vi "XDataNode_OnFontChange.vi"(0 "XRef":T10, 1 "State In":T1 {"Timing"."I/O Scan Engine Mode" max=255 format="%#.0f"; "Timing"."Assigned CPU" min=-2 max=255 format="%#.0f"}) -> (14 "Reply":T8, 15 "State Out":T1 {"Timing"."I/O Scan Engine Mode" max=255 format="%#.0f"; "Timing"."Assigned CPU" min=-2 max=255 format="%#.0f"})   [LabVIEW 2017, in "XDataNode.xnode"]
uses:
  XDataNode.xnode
  XNodeXNodeRef.ctl
  XDataNode.ctl
  timing_clust.ctl
  nitl_modes.ctl
  wakeup.ctl
  TermInfo.ctl
  nitl_TargetSpecificData.ctl
  DN_Type.ctl
  XNodeStringArray.ctl
  XNodeString.ctl
  ReplySet.ctl
  NI_XNodeSupport.lvlib
  XDNodeRunTimeDep.lvlib
panel:
  # "Expected End [f-1]"
  # "Actual End [f-1]"
  # "Finished Late? [f-1]"
  # "Expected End [i-1]"
  # "Actual End [i-1]"
  # "Finished Late? [i-1]"
  # "Exp.Iter.Start"
  # "Act.Iter.Start"
  # "Exp.Frm.Start"
  # "Act.Frm.Start"
  # "Source Name"
  # "Loop/Sequence Name"
  # "Period"
  # "Deadline"
  # "Offset"
  # "Start"
  # "Priority"
  # "Timeout"
  # "Mode"
  # "Wakeup Reason"
  # "Error"
  # "Source Type"
  # "2nd.Src.Type"
  # "Global End Time"
  # "Global Start Time"
  # "Frame Duration"
  # "Iteration Duration"
  # "Assigned CPU"
  # "I/O Scan Engine Mode"
  # "Expected End [f-1]"
  # "Actual End [f-1]"
  # "Finished Late? [f-1]"
  # "Expected End [i-1]"
  # "Actual End [i-1]"
  # "Finished Late? [i-1]"
  # "Exp.Iter.Start"
  # "Act.Iter.Start"
  # "Exp.Frm.Start"
  # "Act.Frm.Start"
  # "Source Name"
  # "Loop/Sequence Name"
  # "Period"
  # "Deadline"
  # "Offset"
  # "Start"
  # "Priority"
  # "Timeout"
  # "Mode"
  # "Wakeup Reason"
  # "Error"
  # "Source Type"
  # "2nd.Src.Type"
  # "Global End Time"
  # "Global Start Time"
  # "Frame Duration"
  # "Iteration Duration"
  # "Assigned CPU"
  # "I/O Scan Engine Mode"
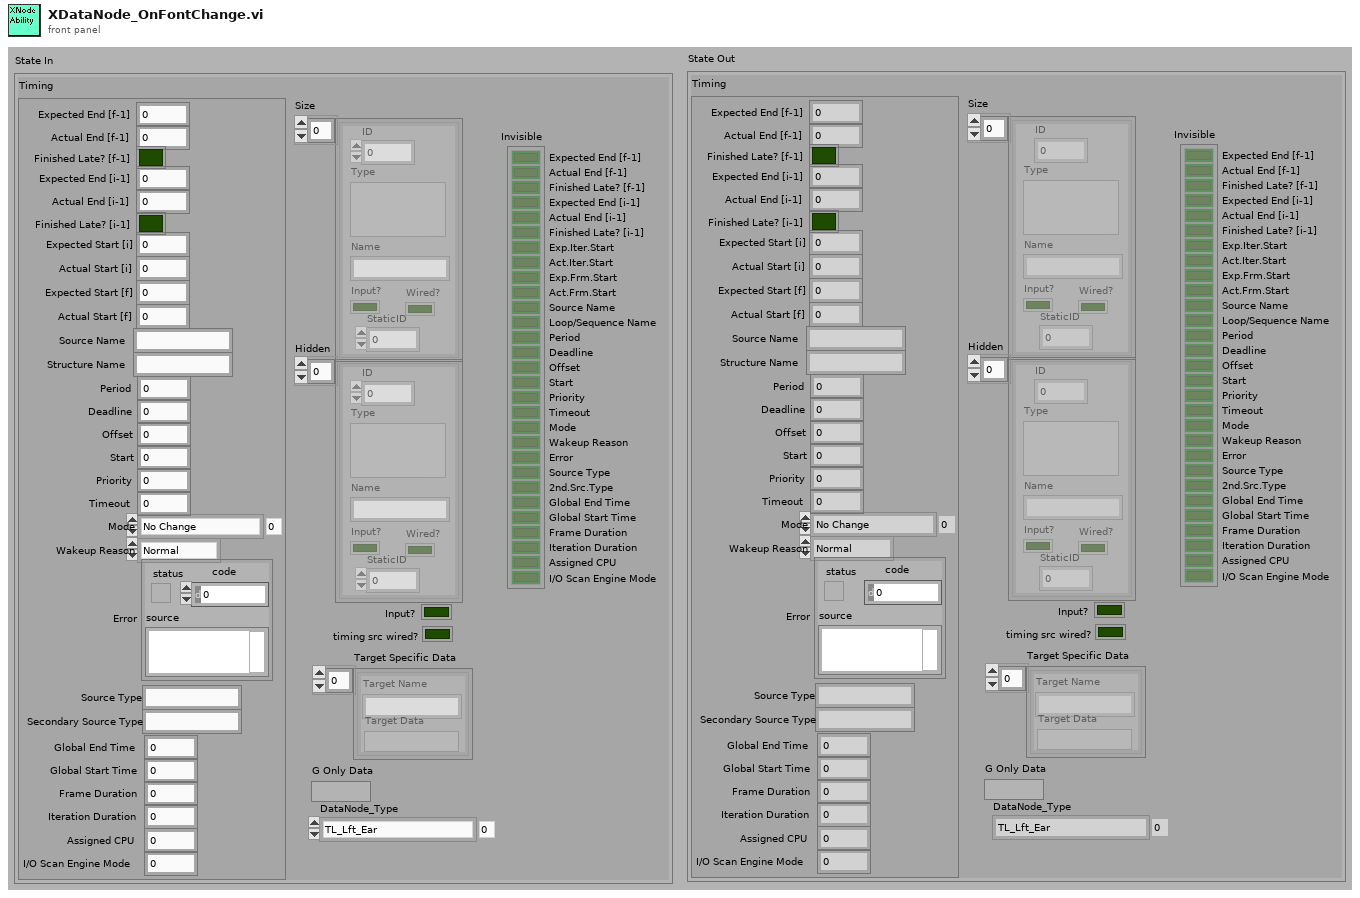
[diagram p1: front panel]
types:
  T1 = typedef "XDataNode.xnode/XDataNode.ctl" = cluster{"Timing":T2, "Size":T5[], "Hidden":T5[], "Invisible":bool[], "Input?":bool, "timing src wired?":bool, "Target Specific Data":T6[], "G Only Data":variant, "DataNode_Type":T7}
  T2 = typedef "XDNodeRunTimeDep.lvlib/timing_clust.ctl" = cluster{"Expected End [f-1]":u64, "Actual End [f-1]":u64, "Finished Late? [f-1]":bool, "Expected End [i-1]":u64, "Actual End [i-1]":u64, "Finished Late? [i-1]":bool, "Expected Start [i]":u64, "Actual Start [i]":u64, "Expected Start [f]":u64, "Actual Start [f]":u64, "Source Name":string, "Structure Name":string, "Period":i64, "Deadline":i64, "Offset":i64, "Start":i64, "Priority":i32, "Timeout":i32, "Mode":T3, "Wakeup Reason":T4, "Error":errorcluster, "Source Type":string, "Secondary Source Type":string, "Global End Time":u64, "Global Start Time":u64, "Frame Duration":u64, "Iteration Duration":u64, "Assigned CPU":i32, "I/O Scan Engine Mode":u32}
  T3 = typedef "XDNodeRunTimeDep.lvlib/nitl_modes.ctl" = enum32{"No Change", "Process missed periods, maintain original phase", "Discard missed periods, maintain original phase", "Process missed periods, ignore original phase", "Discard missed periods, ignore original phase"}
  T4 = typedef "XDNodeRunTimeDep.lvlib/wakeup.ctl" = enum32{"Normal", "Aborted", "Asynchronous wakeup", "Timing source error", "Timed loop error", "Timeout"}
  T5 = typedef "XDataNode.xnode/TermInfo.ctl" = cluster{"ID":i32, "Wired?":bool, "Type":variant, "Name":string, "Input?":bool, "StaticID":i32}
  T6 = typedef "XDataNode.xnode/nitl_TargetSpecificData.ctl" = cluster{"Target Name":string, "Target Data":variant}
  T7 = typedef "XDataNode.xnode/DN_Type.ctl" = enum32{"TL_Lft_Ear", "TL_Rt_Ear", "TL_Lft_Dn", "TL_Rt_Dn", "TS_Lft_Ear", "TS_Rt_Ear", "TS_1stFrame_Lft_Dn", "TS_Lft_Dn", "TS_LastFrame_Rt_Dn", "TS_Rt_Dn", "TL_TS_Lft_Ear", "TL_TS_Rt_Ear", "TL_TS_Lft_Dn", "TL_TS_Rt_Dn", "TL_TS_1stFrame_Lft_Dn", "TL_TS_LastFrame_Rt_Dn"}
  T8 = typedef "NI_XNodeSupport.lvlib/XNodeStringArray.ctl" = T9[]
  T9 = typedef "NI_XNodeSupport.lvlib/XNodeString.ctl" = string
  T10 = typedef "NI_XNodeSupport.lvlib/XNodeXNodeRef.ctl" = refnum<vi>
  T11 = typedef "XDataNode.xnode/ReplySet.ctl" = u16
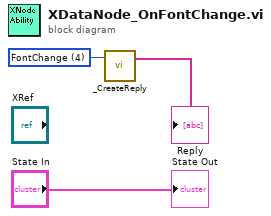
[diagram p0: block diagram]
diagram:
  w1 = T11 4 items=["FullUpdate", "RefeeChanged", "AdaptToInputs", "Refresh", "FontChange"] ("Ring")
  n1 = call "_CreateReply.vi"("Ring"=w1) -> ("Reply"=→"Reply":string[])  [unwired: 2 in]
  "State Out" <- "State In"
